vi "Transmit and Receive with IRIG Time.vi"() -> ()   [LabVIEW 2019]
doc: "This example opens the specified card and core. The provided XML Configuration\nbuilds a transmit schedule using explicit message timing, configures a receive\nchannel and enables the self-test wraparound and filters are set to receive the messages.\nThe hardware time is seeded with the system time using the IRIG. The Airspeed Label \nBlock and the IRIG time structures are displayed."
uses:
  <instrlib>/BTI429Lib/Public/Controls/429 Message Fields.ctl
  <instrlib>/BTICardLib/Public/Controls/IRIG Time.ctl
  <instrlib>/BTICardLib/Public/Controls/Timer Format.ctl
  <instrlib>/BTICardLib/Public/Controls/Timer Resolution.ctl
  <instrlib>/BTICardLib/Private/Initialize By Card Number and Core Number.vi
  <instrlib>/BTICardLib/Private/Configure Core From XML.vi
  <instrlib>/BTI429Lib/Private/Tx/Configure/Configure Tx Channel From XML.vi
  <instrlib>/BTI429Lib/Private/Rx/Configure/Configure Rx Channel From XML.vi
  <instrlib>/BTI429Lib/Private/Rx/Configure/Get Rx Label Handle Name.vi
  <instrlib>/BTI429Lib/Private/Core/Action-Status/Start All Channels.vi
  <instrlib>/BTICardLib/Private/Timing/Utility/Convert Binary Timetag To IRIG Time US.vi
  <instrlib>/BTICardLib/Private/Timing/Utility/Convert Binary Timetag To IRIG Time NS.vi
  <instrlib>/BTICardLib/Private/Timing/Utility/Get IRIG Hours.vi
  <instrlib>/BTICardLib/Private/Timing/Utility/Get IRIG Minutes.vi
  <instrlib>/BTICardLib/Private/Timing/Utility/Get IRIG Seconds.vi
  <instrlib>/BTICardLib/Private/Timing/Utility/Get IRIG Milliseconds.vi
  <instrlib>/BTICardLib/Private/Timing/Utility/Get IRIG Microseconds.vi
  <instrlib>/BTI429Lib/Private/Core/Action-Status/Stop All Channels.vi
  <instrlib>/BTICardLib/BTICardLV.lvlib
  <instrlib>/BTI429Lib/BTI429LV.lvlib
panel:
  out "time":T1
  out "core number":i32
  out "tx channel number":i32
  out "rx channel number":i32
  in  "Rx Channel XML Configuration File Name":string="Channel Config Rx.xml"
  out "Airspeed":T2 {"speed" items=["CHSPEED429_LOW", "CHSPEED429_HIGH"]; "msgdata" format="%08x"; "timetagh" format="%08x"; "timetag_hitcount" format="%08x"; "maxtime_elapsetime" format="%08x"; "mintime" format="%08x"; "paramflag" format="%04x"}
  in  "Tx Channel XML Configuration File Name":string="Channel Config Tx.xml"
  in  "Core XML Configuration File Name":string="Core Config.xml"
  in  "Card Number":i32
  in  "stop":bool
  out "error out":errorcluster
  # "ARINC 429: Transmit and Receive with IRIG Time"
  # "©2016 Astronics Ballard Technology"
  # "This example opens the specified card and core. The provided XML Configuration\nbuilds a transmit schedule using explicit message timing, configures a receive\nchannel and enables the self-test wraparound and filters are set to receive the messages.\nThe hardware time is seeded with the system time using the IRIG. The Airspeed Label \nBlock and the IRIG time structures are displayed."
  # "Always Stop the card\nand Close the card when\ndone. Otherwise, the hardware\ncontinues to operate."
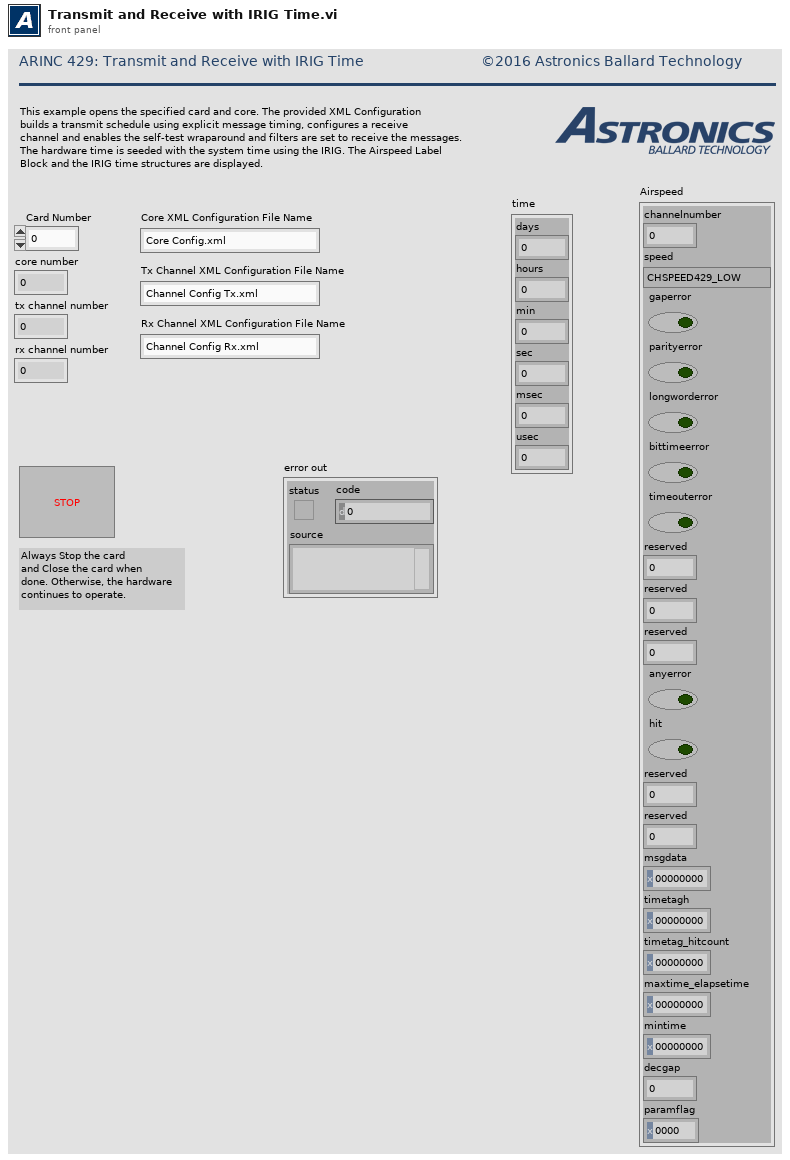
[diagram p1: front panel]
types:
  T1 = typedef "BTICardLV.lvlib/IRIG Time.ctl" = cluster{"days":u16, "hours":u16, "min":u16, "sec":u16, "msec":u16, "usec":u16}
  T2 = typedef "BTI429LV.lvlib/429 Message Fields.ctl" = cluster{"channelnumber":i32, "speed":u32, "gaperror":bool, "parityerror":bool, "longworderror":bool, "bittimeerror":bool, "timeouterror":bool, "reserved":i8, "reserved":i8, "reserved":i8, "anyerror":bool, "hit":bool, "reserved":i8, "reserved":i8, "msgdata":u32, "timetagh":u32, "timetag_hitcount":u32, "maxtime_elapsetime":u32, "mintime":u32, "decgap":u16, "paramflag":u16}
  T3 = typedef "BTICardLV.lvlib/Timer Resolution.ctl" = u32
  T4 = typedef "BTICardLV.lvlib/Timer Format.ctl" = u32
  T5 = typedef "LVDateTimeRec.ctl" = cluster{"fractional second":dbl, "second":i32, "minute":i32, "hour":i32, "day of month":i32, "month":i32, "year":i32, "day of week":i32, "day of year":i32, "DST":i32}
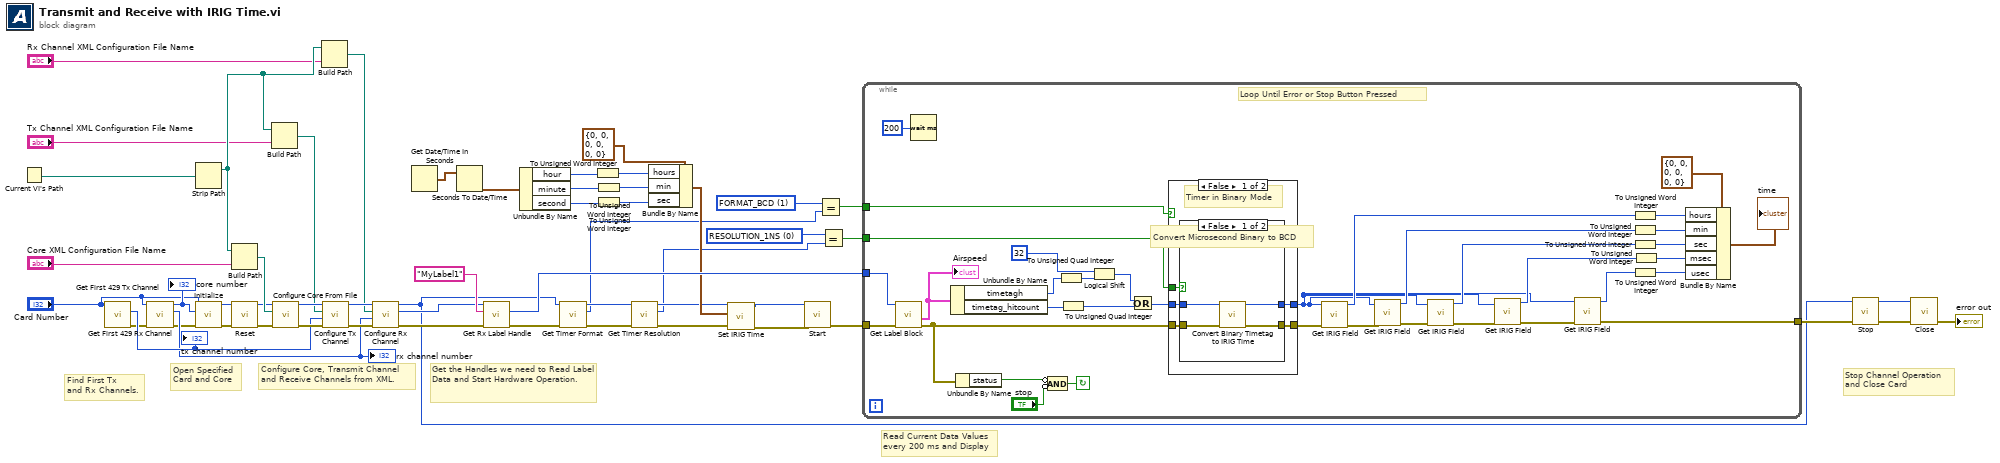
[diagram p0: block diagram]
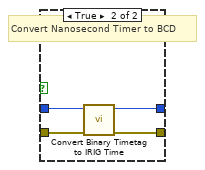
[diagram p2: hidden frame]
diagram:
  w5 = T3 0 items=["RESOLUTION_1NS", "RESOLUTION_1US"] ("resolution")
  w4 = T4 1 items=["FORMAT_BINARY", "FORMAT_BCD"] ("format")
  # "Read Current Data Values\nevery 200 ms and Display"
  # "Find First Tx \nand Rx Channels."
  # "Stop Channel Operation\nand Close Card"
  # "Get the Handles we need to Read Label Data and Start Hardware Operation."
  # "Configure Core, Transmit Channel\nand Receive Channels from XML."
  # "Open Specified\nCard and Core"
  n1 = Current VI's Path() -> (path=w47:path)
  n2 = call "Get First 429 Tx Channel.vi"("Card Number"="Card Number") -> ("error out"=w28:errorcluster, "Channel Number"=w30:i32)  [unwired: 8 in, 1 out]
  "tx channel number" <- w30
  n3 = call "Get First 429 Rx Channel.vi"("error in (no error)"=w28, "Card Number"="Card Number") -> ("error out"=w27:errorcluster, "Channel Number"=w29:i32, "Core Number"=w32:i32)  [unwired: 7 in]
  "rx channel number" <- w29
  "core number" <- w32
  n4 = Strip Path(path=w47) -> (stripped path=w42:path)  [unwired: 1 out]
  n5 = call-poly <instrlib>:"Initialize.vi"("error in (no error)"=w27, "core number"=w32, "card number"="Card Number") -> ("error out"=w34:errorcluster, "core handle out"=w33:u64)  [unwired: 7 in]
  n6 = Build Path(base path=w42, name or relative path="Core XML Configuration File Name") -> (appended path=w43:path)
  n7 = call <instrlib>:"Reset.vi"("error in (no error)"=w34, "core handle in"=w33) -> ("error out"=w35:errorcluster, "core handle out"=w36:u64)  [unwired: 8 in]
  n8 = Build Path(base path=w42, name or relative path="Tx Channel XML Configuration File Name") -> (appended path=w38:path)
  n9 = call-poly <instrlib>:"Configure Core From File.vi"("error in (no error)"=w35, "configuration file path"=w43, "core handle in"=w36) -> ("error out"=w55:errorcluster, "core handle out"=w39:u64)  [unwired: 7 in]
  n10 = Build Path(base path=w42, name or relative path="Rx Channel XML Configuration File Name") -> (appended path=w40:path)
  n11 = call-poly <instrlib>:"Configure Tx Channel.vi"("error in (no error)"=w55, "channel number in"=w30, "configuration file path"=w38, "core handle in"=w39) -> ("error out"=w44:errorcluster, "core handle out"=w45:u64)  [unwired: 5 in, 1 out]
  n12 = call-poly <instrlib>:"Configure Rx Channel.vi"("error in (no error)"=w44, "channel number in"=w29, "configuration file path"=w40, "core handle in"=w45) -> ("error out"=w16:errorcluster, "channel handle out"=w17:u64, "core handle out"=w9:u64)  [unwired: 5 in]
  n13 = Get Date/Time In Seconds() -> (seconds since 1Jan1904=w25:timestamp)
  n14 = Seconds To Date/Time(time stamp (now)=w25) -> (date time rec=w24:T5)  [unwired: 1 in]
  n15 = call-poly <instrlib>:"Get Rx Label Handle.vi"("error in (no error)"=w16, "label name"="MyLabel1", "channel handle in"=w17) -> ("error out"=w12:errorcluster, "label handle out"=w49:u64)  [unwired: 6 in, 1 out]
  n16 = Unbundle By Name(w24) -> ("hour"=w19:i32, "minute"=w21:i32, "second"=w23:i32)
  n17 = call <instrlib>:"Get Timer Format.vi"("error in (no error)"=w12, "core handle in"=w9) -> ("error out"=w11:errorcluster, "format"=w3:T4, "core handle out"=w8:u64)  [unwired: 7 in]
  n18 = To Unsigned Word Integer(number=w19) -> (unsigned 16bit integer=w18:u16)
  n19 = To Unsigned Word Integer(number=w21) -> (unsigned 16bit integer=w20:u16)
  n20 = To Unsigned Word Integer(number=w23) -> (unsigned 16bit integer=w22:u16)
  n21 = call <instrlib>:"Get Timer Resolution.vi"("error in (no error)"=w11, "core handle in"=w8) -> ("error out"=w10:errorcluster, "resolution"=w6:T3, "core handle out"=w7:u64)  [unwired: 7 in]
  n22 = Bundle By Name(cluster=T1 {"days"=0, "hours"=0, "min"=0, "sec"=0, "msec"=0, "usec"=0} ("time"), "hours"=w18, "min"=w20, "sec"=w22) -> (w15:T1)
  n23 = call <instrlib>:"Set IRIG Time.vi"("error in (no error)"=w10, "time"=w15, "core handle in"=w7) -> ("error out"=w14:errorcluster, "core handle out"=w13:u64)  [unwired: 7 in]
  n24 = call-poly <instrlib>:"Start.vi"("error in (no error)"=w14, "core handle in"=w13) -> ("error out"=w50:errorcluster)  [unwired: 8 in, 1 out]
  n25 = Equal?(x=w4, y=w3) -> (x = y?=w2:bool)
  n26 = Equal?(x=w5, y=w6) -> (x = y?=w1:bool)
  n27 = while {
    tunnel: [w64] -> w51
    tunnel: w50 -> [w87]
    tunnel: w49 -> [w88]
    tunnel: w2 -> [w59]
    tunnel: w1 -> [w58]
    stop <- w90 continue-if-true
    # "Loop Until Error or Stop Button Pressed"
    n28 = call <instrlib>:"Get Label Block.vi"("error in (no error)"=w87, "label handle in"=w88) -> ("error out"=w62:errorcluster, "value"=w57:T2)  [unwired: 6 in, 2 out]
    "Airspeed" <- w57
    n29 = Wait (ms)(milliseconds to wait=u32 200) -> ()  [unwired: 1 out]
    n30 = Unbundle By Name(w57) -> ("timetagh"=w68:u32, "timetag_hitcount"=w67:u32)
    n31 = Unbundle By Name(w62) -> ("status"=w89:bool)
    n32 = Compound Arithmetic op=AND(invert w89, invert "stop") -> (w90:bool)
    n33 = To Unsigned Quad Integer(1:w68) -> (0:w69:u64)
    n34 = To Unsigned Quad Integer(1:w67) -> (0:w66:u64)
    n35 = Logical Shift(y=32, x=w69) -> (x << y=w65:u64)
    n36 = Or(x=w65, y=w66) -> (x .or. y?=w61:u64)
    n37 = case shown="False" w59 {
      tunnel: [w96 w106] -> w63
      tunnel: w62 -> [w95 w106]
      tunnel: w61 -> [w94 w105]
      tunnel: [w93 w105] -> w60
      tunnel: w58 -> [w92 _]
      frame False {
        # "Timer in Binary Mode"
        n38 = case shown="False" w92 {
          tunnel: [w100 w103] -> w96
          tunnel: w95 -> [w99 w104]
          tunnel: w94 -> [w98 w101]
          tunnel: [w97 w102] -> w93
          frame False {
            # "Convert Microsecond Binary to BCD"
            n39 = call-poly <instrlib>:"Convert Binary Timetag to IRIG Time.vi"("error in (no error)"=w99, "binary time us"=w98) -> ("error out"=w100:errorcluster, "IRIG time"=w97:u64)  [unwired: 8 in]
          }
          frame True {
            # "Convert Nanosecond Timer to BCD"
            n40 = call-poly <instrlib>:"Convert Binary Timetag to IRIG Time.vi"("error in (no error)"=w104, "binary time ns"=w101) -> ("error out"=w103:errorcluster, "IRIG time"=w102:u64)  [unwired: 8 in]
          }
        }
      }
      frame True {
        # "Timer in BCD Mode"
      }
    }
    n41 = call-poly <instrlib>:"Get IRIG Field.vi"("error in (no error)"=w63, "IRIG time"=w60) -> ("error out"=w82:errorcluster, "hours"=w84:u32)  [unwired: 8 in]
    n42 = call-poly <instrlib>:"Get IRIG Field.vi"("error in (no error)"=w82, "IRIG time"=w60) -> ("error out"=w81:errorcluster, "minutes"=w78:u32)  [unwired: 8 in]
    n43 = call-poly <instrlib>:"Get IRIG Field.vi"("error in (no error)"=w81, "IRIG time"=w60) -> ("seconds"=w80:errorcluster, "function return"=w77:u32)  [unwired: 8 in]
    n44 = call-poly <instrlib>:"Get IRIG Field.vi"("error in (no error)"=w80, "IRIG time"=w60) -> ("error out"=w79:errorcluster, "milliseconds"=w76:u32)  [unwired: 8 in]
    n45 = call-poly <instrlib>:"Get IRIG Field.vi"("error in (no error)"=w79, "IRIG time"=w60) -> ("error out"=w64:errorcluster, "microseconds"=w75:u32)  [unwired: 8 in]
    n46 = To Unsigned Word Integer(number=w84) -> (unsigned 16bit integer=w83:u16)
    n47 = To Unsigned Word Integer(number=w78) -> (unsigned 16bit integer=w71:u16)
    n48 = To Unsigned Word Integer(number=w77) -> (unsigned 16bit integer=w72:u16)
    n49 = To Unsigned Word Integer(number=w75) -> (unsigned 16bit integer=w74:u16)
    n50 = To Unsigned Word Integer(number=w76) -> (unsigned 16bit integer=w73:u16)
    n51 = Bundle By Name(cluster=T1 {"days"=0, "hours"=0, "min"=0, "sec"=0, "msec"=0, "usec"=0} ("time"), "hours"=w83, "min"=w71, "sec"=w72, "msec"=w73, "usec"=w74) -> (→"time":T1)
  }
  n52 = call-poly <instrlib>:"Stop.vi"("error in (no error)"=w51, "core handle in"=w9) -> ("error out"=w54:errorcluster, "core handle out"=w52:u64)  [unwired: 8 in]
  n53 = call <instrlib>:"Close.vi"("error in (no error)"=w54, "core handle in"=w52) -> ("error out"=→"error out":errorcluster)  [unwired: 8 in, 1 out]
